vi "write_controller_file.vi"(6 "5V reg":cluster{dbl, dbl}, 7 "3.3V reg":cluster{dbl, dbl}, 9 "BUS":cluster{dbl, dbl, dbl}, 10 "minutes":dbl, 11 "controller file":path) -> ()   [LabVIEW 2019]
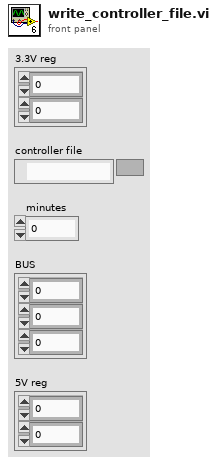
[diagram p1: front panel]
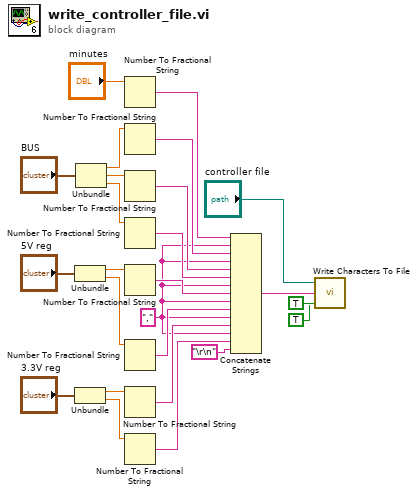
[diagram p0: block diagram]
diagram:
  w4 = "," ("string")
  n1 = Unbundle("5V reg") -> (w22:dbl, w8:dbl)
  n2 = Unbundle("3.3V reg") -> (w6:dbl, w3:dbl)
  n3 = Unbundle("BUS") -> (w13:dbl, w14:dbl, w15:dbl)
  n4 = Number To Fractional String(number="minutes") -> (F-format string=w16:string)  [unwired: 3 in]
  n5 = Number To Fractional String(number=w13) -> (F-format string=w17:string)  [unwired: 3 in]
  n6 = Number To Fractional String(number=w14) -> (F-format string=w18:string)  [unwired: 3 in]
  n7 = Number To Fractional String(number=w15) -> (F-format string=w19:string)  [unwired: 3 in]
  n8 = Number To Fractional String(number=w22) -> (F-format string=w23:string)  [unwired: 3 in]
  n9 = Number To Fractional String(number=w8) -> (F-format string=w7:string)  [unwired: 3 in]
  n10 = Number To Fractional String(number=w6) -> (F-format string=w5:string)  [unwired: 3 in]
  n11 = Number To Fractional String(number=w3) -> (F-format string=w2:string)  [unwired: 3 in]
  n12 = Concatenate Strings(w16, w4, w17, w4, w18, w19, w4, w23, w4, w7, w4, w5, w4, w2, "\r\n") -> (w24:string)
  n13 = call <vilib>:"Write Characters To File.vi"("convert eol? (no:F)"=TRUE, "append to file? (new file:F)"=TRUE, "character string"=w24, "file path (dialog if empty)"="controller file") -> ()  [unwired: 1 in, 1 out]
